vi "FTW-Example-SlasdClient-Core-Initialize.vi"(0 "Initialization Sequence":string, 5 "FTW Actor Instance Configuration":string, 11 "error in (no error)":errorcluster) -> (4 "Actor Template-Core out":refnum<class "FTW-Example-SlasdClient-Core.lvclass">, 6 "Incoming Requests":refnum<event-registration>, 8 "SLASD Subscription":refnum<event-registration>, 15 "error out":errorcluster)   [LabVIEW 2013, in "FTW-Example-SlasdClient-Core.lvclass"]
uses:
  FTW-Example-SlasdClient-Core.lvclass
  source/actor/Message/Request/FTW-Message-IncomingRequest.lvclass
  source/actor/Message/Base/FTW-Message.lvclass
  FTW-Example-SlasdClient-Core.lvclass/FTW-Example-SlasdClient-Core.ctl
  source/Reflection/FTW-Reflection-Type.vi
  source/JSON/FTW-JSON-Core-LibraryFilepath.vi
  source/JSON/FTW-JSON-Core-GetFlattenedValue.vi
  source/JSON/FTW-JSON-Core-LibraryError.vi
  source/CodeGen/JSON Deserialize/FTW-JSON-Deserialize.xnode
  SLASD/FTW-Example-SLASD.lvclass
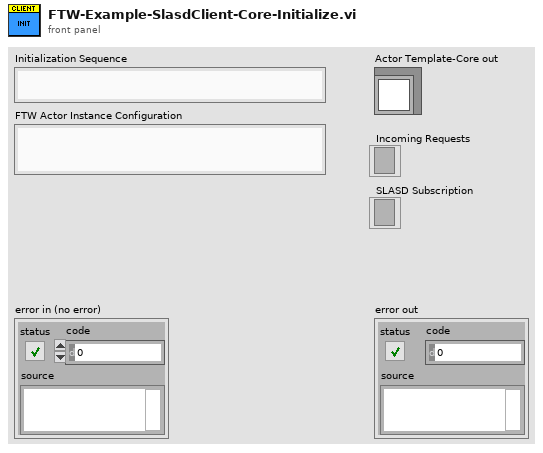
[diagram p1: front panel]
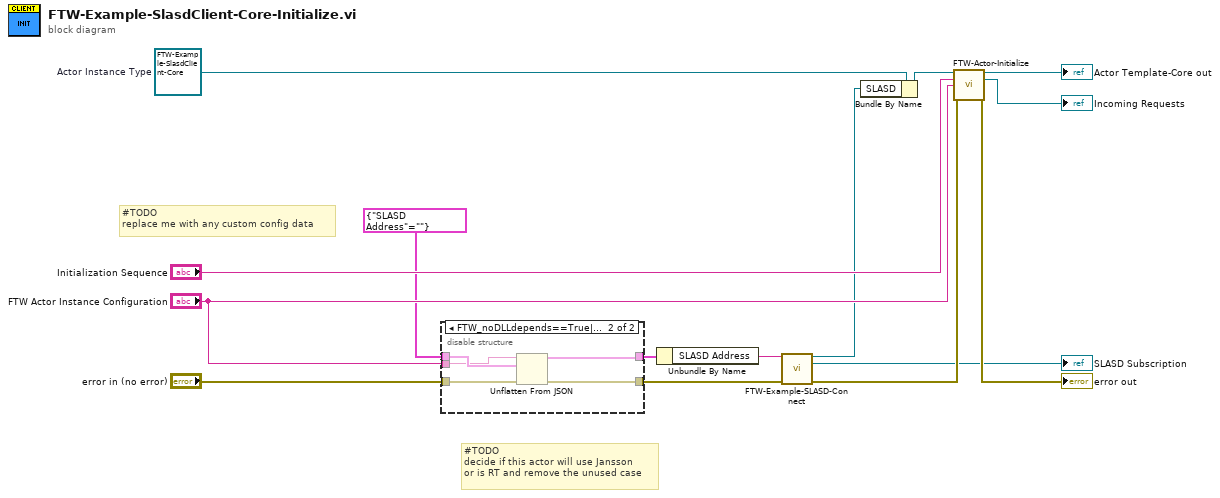
[diagram p0: block diagram]
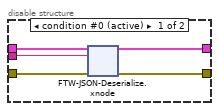
[diagram p2: hidden frame]
diagram:
  w6 = refnum<class "FTW-Example-SlasdClient-Core.lvclass"> refnum  # Actor Instance Type
  # "#TODO\ndecide if this actor will use Jansson\nor is RT and remove the unused case"
  # "#TODO\nreplace me with any custom config data"
  n1 = disable-structure shown="FTW_noDLLdepends==True||TARGET_TYPE==RT" {
    disable-tunnel: "error in (no error)" -> [w20 w59]
    disable-tunnel: [w19 w58] -> w10
    disable-tunnel: "FTW Actor Instance Configuration" -> [w18 w56]
    disable-tunnel: cluster{"SLASD Address":string} {"SLASD Address"=""} ("Type and Defaults") -> [w17 w57]
    disable-tunnel: [w16 w55] -> w7
    frame condition #0 (active) {
      n2 = xnode "FTW-JSON-Deserialize.xnode"("Type and Defaults"=w17, "JSON String"=w18, "error in"=w20) -> ("Values"=w16:cluster{"SLASD Address":string}, "error out"=w19:errorcluster)
    }
    frame condition #1 {
      n3 = Unflatten From JSON(JSON string=w56, type and defaults=w57, error in (no error)=w59) -> (value=w55:cluster{"SLASD Address":string}, error out=w58:errorcluster)  [unwired: 4 in]
    }
  }
  n4 = Unbundle By Name(w7) -> ("SLASD Address"=w4:string)
  n5 = call "FTW-Example-SLASD-Connect.vi"("IP Address"=w4, "error in"=w10) -> ("FTW Actor Connector"=w2:refnum<class "FTW-Example-SLASD.lvclass">, "Subscription Registration Refnum"=→"SLASD Subscription":refnum<event-registration>, "error out"=w5:errorcluster)  [unwired: 11 in]
  n6 = Bundle By Name(cluster=w6, "SLASD"=w2) -> (w3:refnum<class "FTW-Example-SlasdClient-Core.lvclass">)
  n7 = call-dynamic "FTW-Actor-Initialize.vi"("FTW Actor Instance Type"=w3, "Initialization Job Sequence"="Initialization Sequence", "Actor Instance Configuration"="FTW Actor Instance Configuration", "error in"=w5) -> ("FTW Actor Instance"=→"Actor Template-Core out":refnum<class "FTW-Example-SlasdClient-Core.lvclass">, "Incoming Requests"=→"Incoming Requests":refnum<event-registration>, "error out"=→"error out":errorcluster)  [unwired: 8 in, 1 out]
